vi "test_avi_save.vi"() -> ()   [LabVIEW 2019]
uses:
  <vilib>/userDefined/High Color/IMAQdx.ctl
  <vilib>/vision/driver/NI_Vision_Acquisition_Software.lvlib
panel:
  in  "index":i32=2
  out "Codec Names":string[](array[string])=["", "", "Microsoft Video 1", "FF Video Codec 1 (FFV1) (NI Vision)", "Motion JPEG (NI Vision)", "VP8 (NI Vision)", "VP9 (NI Vision)", "Y800 Uncompressed Grey Scale (NI Vision)", "YUV 4:2:0 Planar (NI Vision)"]
  in  "AVI Path":path=path "C:/AGV/Log/08/pusan_track_c922.avi"
  in  "Session In":T1="cam1"
  in  "Frames Per Second for AVI Playback":u32=10
  in  "Stop":bool
  out "Image":T2(plugin-control)
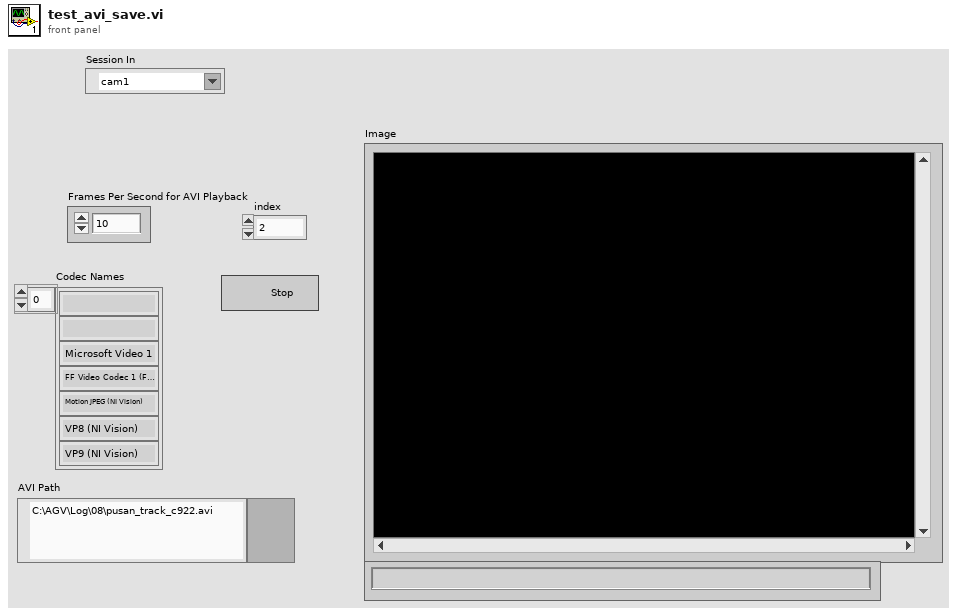
[diagram p1: front panel]
types:
  T1 = typedef "IMAQdx.ctl" = refnum<k21>
  T2 = typedef "IMAQ Image.ctl" = refnum<image>
  T3 = typedef "IMAQ AVI2 Refnum.ctl" = refnum<k20>
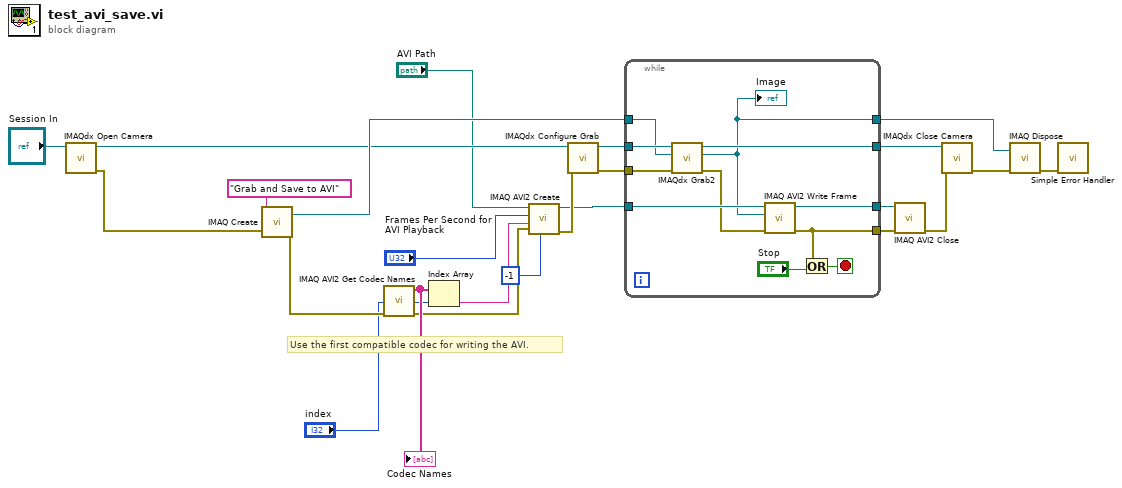
[diagram p0: block diagram]
diagram:
  # "Use the first compatible codec for writing the AVI."
  n1 = call <vilib>:"IMAQdx Open Camera.vi"("Session In"="Session In") -> ("error out"=w5:errorcluster, "Session Out"=w6:T1)  [unwired: 9 in]
  n2 = call "IMAQ Create"("Image Name"="Grab and Save to AVI", "error in (no error)"=w5) -> ("New Image"=w24:T2, "error out"=w9:errorcluster)  [unwired: 2 in, 1 out]
  n3 = call "IMAQ AVI2 Get Codec Names"("error in (no error)"=w9) -> ("error out"=w7:errorcluster, "Codec Names"=w10:string[])  [unwired: 9 in]
  "Codec Names" <- w10
  n4 = Index Array(array=w10, index="index") -> (element=w8:string)
  n5 = call "IMAQ AVI2 Create"("Quality"=-1, "error in (no error)"=w7, "Codec"=w8, "Frames Per Second"="Frames Per Second for AVI Playback", "AVI Path"="AVI Path") -> ("error out"=w16:errorcluster, "AVI Refnum"=w14:T3)  [unwired: 5 in]
  n6 = call <vilib>:"IMAQdx Configure Grab.vi"("error in"=w16, "Session In"=w6) -> ("error out"=w17:errorcluster, "Session Out"=w18:T1)  [unwired: 8 in]
  n7 = while {
    tunnel: [w30] -> w23
    tunnel: w24 -> [w33]
    tunnel: w18 -> [w34]
    tunnel: w17 -> [w35]
    tunnel: [w26] -> w12
    tunnel: [w27] -> w22
    tunnel: [w25] -> w13
    tunnel: w14 -> [w29]
    stop <- w32 stop-if-true
    n8 = call <vilib>:"IMAQdx Grab2.vi"("error in"=w35, "Image In"=w33, "Session In"=w34) -> ("error out"=w28:errorcluster, "Image Out"=w27:T2, "Session Out"=w30:T1)  [unwired: 5 in, 1 out]
    "Image" <- w27
    n9 = call "IMAQ AVI2 Write Frame"("error in (no error)"=w28, "Image"=w27, "AVI Refnum"=w29) -> ("error out"=w26:errorcluster, "AVI Refnum (duplicate)"=w25:T3)  [unwired: 6 in, 1 out]
    n10 = Or(x=w26, y="Stop") -> (x .or. y?=w32:bool)
  }
  n11 = call "IMAQ AVI2 Close"("error in (no error)"=w12, "AVI Refnum"=w13) -> ("error out"=w11:errorcluster)  [unwired: 9 in]
  n12 = call <vilib>:"IMAQdx Close Camera.vi"("error in"=w11, "Session In"=w23) -> ("error out"=w19:errorcluster)  [unwired: 9 in]
  n13 = call "IMAQ Dispose"("Image"=w22, "error in (no error)"=w19) -> ("error out"=w21:errorcluster)  [unwired: 1 in, 3 out]
  n14 = call <vilib>:"Simple Error Handler.vi"("error in (no error)"=w21) -> ()  [unwired: 1 in, 8 out]
